vi "calculate Qs.vi"(8 "length 2":dbl, 9 "length 1":dbl, 10 "y":dbl, 11 "x":dbl) -> (0 "cosq2 (config 2)":dbl, 1 "cosq2 (config 1)":dbl, 2 "q2 (config 1)":dbl, 3 "q1 (config 1)":dbl, 4 "p1 (for debug":dbl, 5 "a2 (for debug)":dbl, 6 "q2 (config 2)":dbl, 7 "q1 (config 2)":dbl)   [LabVIEW 2023]
panel:
  out "a1 (for debug)":dbl
  out "WRONG q1":dbl
  out "WRONG q2":dbl
  out "WRONG cos q2":dbl
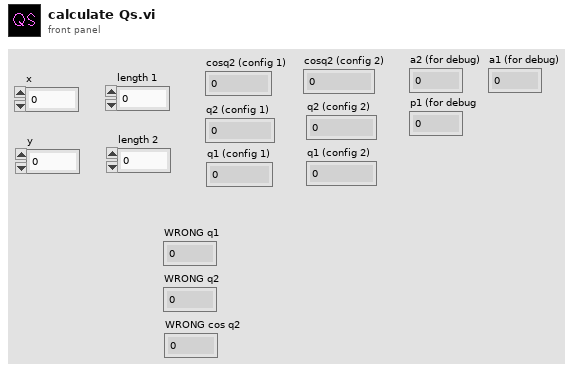
[diagram p1: front panel]
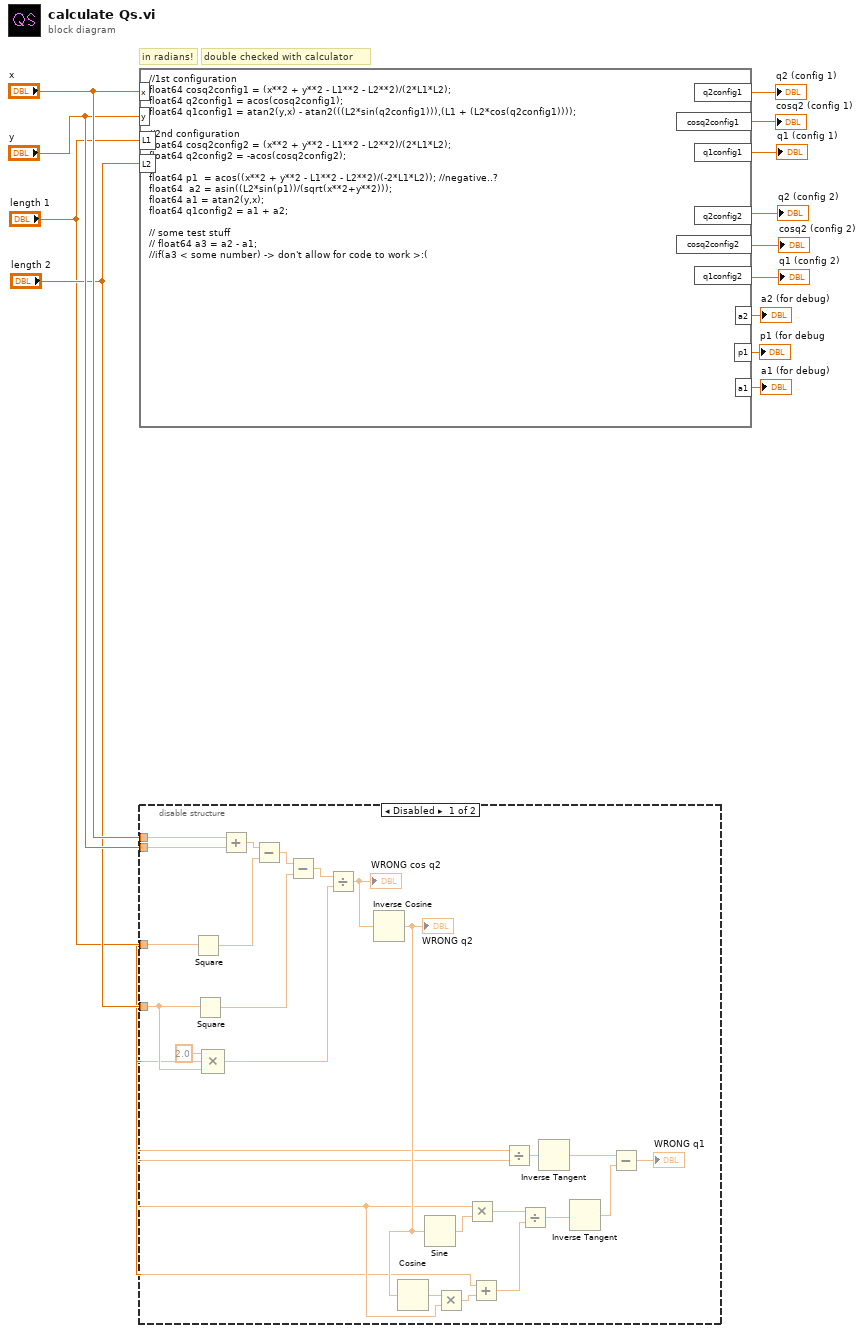
[diagram p0: block diagram]
diagram:
  # "double checked with calculator"
  # "in radians!"
  n1 = formula code="//1st configuration\nfloat64 cosq2config1 = (x**2 + y**2 - L1**2 - L2**2)/(2*L1*L2);\nfloat64 q2config1 = acos(cosq2config1);\nfloat64 q1config1 = atan2(y,x) - atan2(((L2*sin(q2config1))),(L1 + (L2*cos(q2config1))));\n\n//2nd configuration\nfloat64 cosq2config2 = (x**2 + y**2 - L1**2 - L2**2)/(2*L1*L2);\nfloat64 q2config2 = -acos(cosq2config2);\n\nfloat64 p1  = acos((x**2 + y**2 - L1**2 - L2**2)/(-2*L1*L2)); //negative..?\nfloat64  a2 = asin((L2*sin(p1))/(sqrt(x**2+y**2)));\nfloat64 a1 = atan2(y,x);\nfloat64 q1config2 = a1 + a2;\n\n// some test stuff\n// float64 a3 = a2 - a1; \n//if(a3 < some number) -> don't allow for code to work >:("("x"="x", "y"="y", "L1"="length 1", "L2"="length 2") -> ("q2config1"=→"q2 (config 1)":dbl, "cosq2config1"=→"cosq2 (config 1)":dbl, "q1config1"=→"q1 (config 1)":dbl, "cosq2config2"=→"cosq2 (config 2)":dbl, "q2config2"=→"q2 (config 2)":dbl, "q1config2"=→"q1 (config 2)":dbl, "a2"=→"a2 (for debug)":dbl, "p1"=→"p1 (for debug":dbl, "a1"=→"a1 (for debug)":dbl)
  n2 = disable-structure shown="Disabled" {
    disable-tunnel: "x" -> [w17 _]
    disable-tunnel: "y" -> [w16 _]
    disable-tunnel: "length 2" -> [w15 _]
    disable-tunnel: "length 1" -> [w14 _]
    frame Disabled {
      n3 = Square(x=w14) -> (x^2=w35:dbl)
      n4 = Square(x=w15) -> (x^2=w33:dbl)
      n5 = Compound Arithmetic op=MULTIPLY(2.0 ("value"), w14, w15) -> (w30:dbl)
      n6 = Add(x=w17, y=w16) -> (x+y=w36:dbl)
      n7 = Subtract(x=w36, y=w35) -> (x-y=w34:dbl)
      n8 = Subtract(x=w34, y=w33) -> (x-y=w31:dbl)
      n9 = Divide(x=w31, y=w30) -> (x/y=w29:dbl)
      "WRONG cos q2" <- w29
      n10 = Inverse Cosine(1:w29) -> (0:w21:dbl)
      "WRONG q2" <- w21
      n11 = Cosine(x=w21) -> (cos(x)=w23:dbl)
      n12 = Sine(x=w21) -> (sin(x)=w26:dbl)
      n13 = Multiply(x=w23, y=w15) -> (x*y=w22:dbl)
      n14 = Multiply(x=w15, y=w26) -> (x*y=w25:dbl)
      n15 = Add(x=w14, y=w22) -> (x+y=w24:dbl)
      n16 = Divide(x=w16, y=w17) -> (x/y=w28:dbl)
      n17 = Divide(x=w25, y=w24) -> (x/y=w20:dbl)
      n18 = Inverse Tangent(1:w28) -> (0:w27:dbl)
      n19 = Inverse Tangent(1:w20) -> (0:w19:dbl)
      n20 = Subtract(x=w27, y=w19) -> (x-y=→"WRONG q1":dbl)
    }
    frame Enabled {
    }
  }
